vi "dscADCodeToVoltage.vi"(8 "error in":errorcluster, 9 "AD Settings":T1 {"load cal" items=["DO NOT LOAD CAL", "LOAD CAL"]}, 10 "adCode":i16, 11 "board":i16) -> (0 "error out":errorcluster, 1 "Settings Out":T1 {"load cal" items=["DO NOT LOAD CAL", "LOAD CAL"]}, 2 "voltage":dbl, 3 "boardOut":i16)   [LabVIEW 2011, in "Diamond Universal Driver.lvlib"]
doc: "Utility function for converting AD units to voltage based on the AD settings used."
uses:
  Diamond Universal Driver.lvlib
  Controls/dscADSettings.ctl
  Controls/gain.ctl
  Controls/error codes.ctl
  Instruments/WL OPC/Support/dlls/dscud.dll
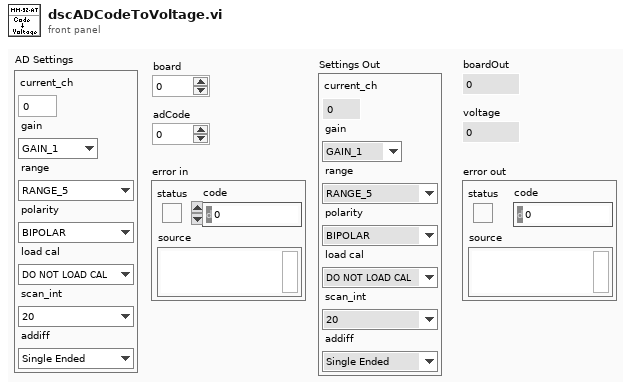
[diagram p1: front panel]
types:
  T1 = typedef "dscADSettings.ctl" = cluster{"current_ch":u8, "gain":T2, "range":enum8{"RANGE_5", "RANGE_10"}, "polarity":enum16{"BIPOLAR", "UNIPOLAR"}, "load cal":u8, "scan_int":enum8{"20", "15", "10", "5", "9", "4"}, "addiff":enum8{"Single Ended", "Differential"}}
  T2 = typedef "gain.ctl" = enum8{"GAIN_1", "GAIN_2", "GAIN_8"}
  T3 = typedef "Diamond Universal Driver.lvlib/error codes.ctl" = enum8{"DE_NONE", "DE_HW_FAILURE", "DE_SW_FAILURE", "DE_HW_NOT_SUPPORTED", "DE_SW_NOT_SUPPORTED", "DE_INVALID_PARM", "DE_ALTERNATE_IN_PROGRESS", "DE_NONE_IN_PROGRESS", "DE_BUFFER_ROLLOVER", "DE_INVALID_ERROR_CODE", "DE_ALREADY_PAUSED", "DE_OVERFLOW", "DE_INVALID_FUNC", "DE_DSCUDH_INVALID", "DE_INVALID_BOARD", "DE_BOARD_LIMIT_REACHED", "DE_BOARD_BUSY", "DE_INVALID_WINDRVR_HANDLE", "DE_INVALID_WINDRVR_VERSION", "DE_BAD_WINDRVR_BOARD_INIT", "DE_OPERATION_TIMED_OUT", "DE_INVALID_WINDRVR_KP", "DE_THREAD_FAILURE"}
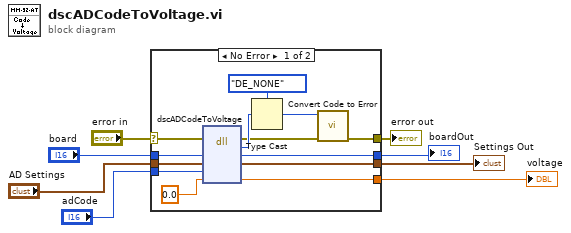
[diagram p0: block diagram]
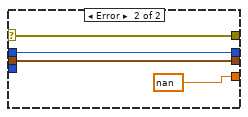
[diagram p2: hidden frame]
diagram:
  n1 = case shown="No Error" "error in" {
    selector: "error in" -> [w18 w25]
    tunnel: "board" -> [w16 w24]
    tunnel: [w15 w24] -> w6
    tunnel: [w14 w25] -> w5
    tunnel: "AD Settings" -> [w13 w23]
    tunnel: "adCode" -> [w12 _]
    tunnel: [w10 sgl nan ("voltage")] -> w2
    tunnel: [w9 w23] -> w1
    frame No Error {
      n2 = dll-call lib="C:/Users/mrichardson/Documents/Web Based Version Control SW/Instruments/WL OPC/Support/dlls/dscud.dll" fn="dscADCodeToVoltage"(error in=w18, "board"=w16, "adSettings"=w13, "adCode"=w12, "voltage"=0.0) -> (error out=w17:errorcluster, "error"=w19:u8, "board"=w15:i16, "adSettings"=w9:T1, "voltage"=w10:dbl)  [unwired: 3 in, 1 out]
      n3 = Type Cast(type=error_codes."DE_NONE" ("error codes"), x=w19) -> (*(type *) &x=w21:T3)
      n4 = call "Convert Code to Error.vi"("error in"=w17, "error codes"=w21) -> ("error out"=w14:errorcluster)  [unwired: 9 in]
    }
    frame Error {
    }
  }
  "boardOut" <- w6
  "error out" <- w5
  "voltage" <- w2
  "Settings Out" <- w1
